vi "Host - Sort Controls.vi"(11 "Controls":refnum<vi>[](array[refnum])) -> (0 "Array":u32[](array[numeric]), 2 "Names":string[](array[string]), 3 "Sorted Ref":refnum<vi>[](array[refnum]))   [LabVIEW 2021]
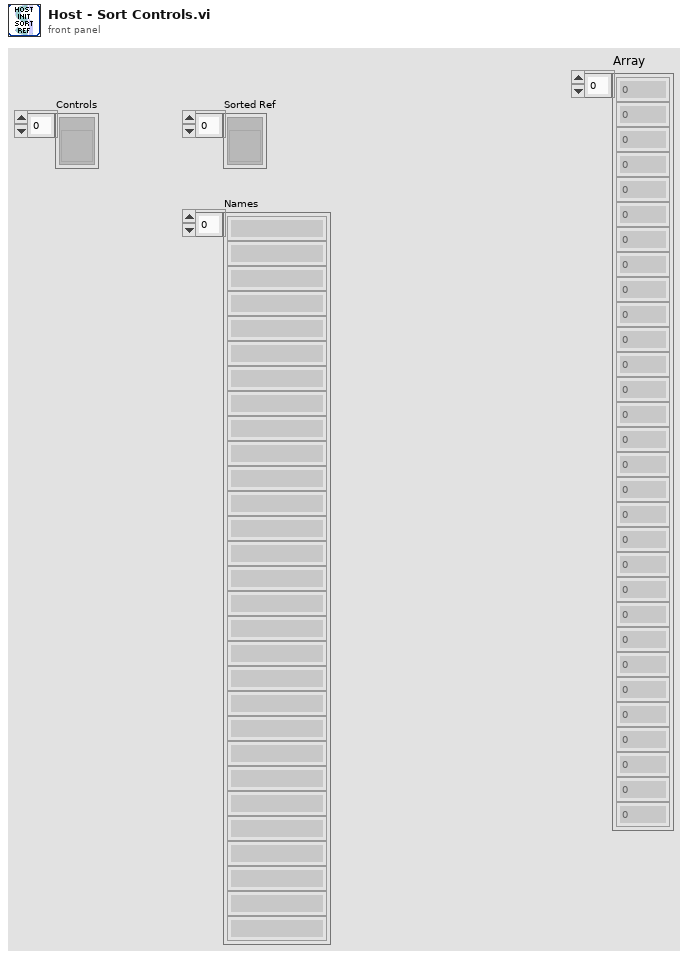
[diagram p1: front panel]
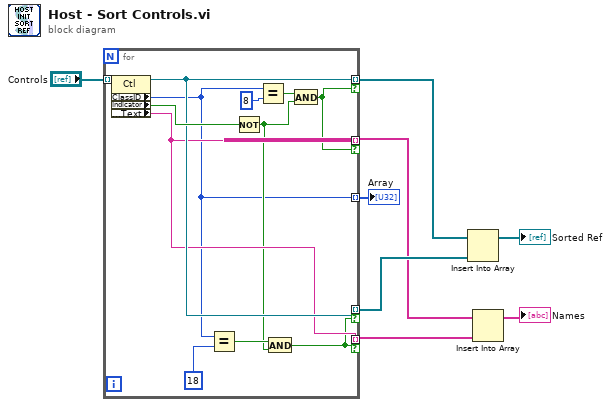
[diagram p0: block diagram]
diagram:
  n1 = for {
    tunnel: [w15] -> w5 mode=indexing if=w17
    tunnel: "Controls" -> [w18] mode=indexing
    tunnel: [w14] -> w3 mode=indexing if=w17
    tunnel: [w15] -> w6 mode=indexing if=w10
    tunnel: [w14] -> w2 mode=indexing if=w10
    tunnel: [w9] -> w7 mode=indexing
    n2 = property class="Ctl"(reference=w18) -> (reference out=w15:refnum<vi>, "ClassID"=w9:u32, "Indicator"=w16:bool, "Label.Text"=w14:string)  [unwired: 1 in, 1 out]
    n3 = Equal?(x=w9, y=u32 18 ("Boolean ClassID")) -> (x = y?=w12:bool)
    n4 = Not(x=w16) -> (.not. x?=w11:bool)
    n5 = Equal?(x=w9, y=u32 8 ("Boolean ClassID")) -> (x = y?=w19:bool)
    n6 = And(x=w12, y=w11) -> (x .and. y?=w10:bool)
    n7 = And(x=w19, y=w11) -> (x .and. y?=w17:bool)
  }
  "Array" <- w7
  n8 = Insert Into Array(array=w5, new element=w6) -> (→"Sorted Ref":refnum<vi>[])  [unwired: 1 in]
  n9 = Insert Into Array(array=w3, new element=w2) -> (→"Names":string[])  [unwired: 1 in]
